vi "Tek_Read.vi"(8 "error in (no error)":errorcluster, 11 "VISA Refnum in":refnum<visa-resource-name>) -> (0 "error out":errorcluster, 1 "range":T1, 2 "Scope":cluster{dbl, dbl, dbl[]}(graph), 3 "VISA Refnum out":refnum<visa-resource-name>)   [LabVIEW 2022 SP3]
panel:
  out "data":dbl[](array[numeric])
  out "YOffset":dbl
  out "XZero":dbl
  out "YZero":dbl
  out "YMult":dbl
  out "XMult":dbl
  out "s/div":dbl
  out "V/div":dbl
  out "array":string[](array[string])
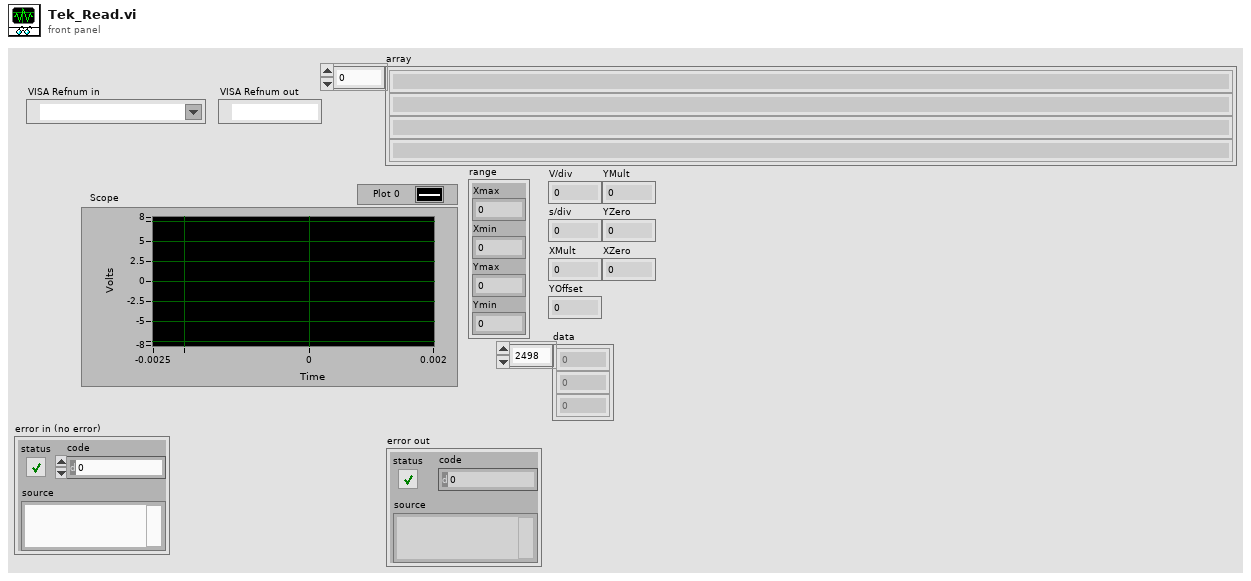
[diagram p1: front panel]
types:
  T1 = cluster{"Xmax":dbl, "Xmin":dbl, "Ymax":dbl, "Ymin":dbl}
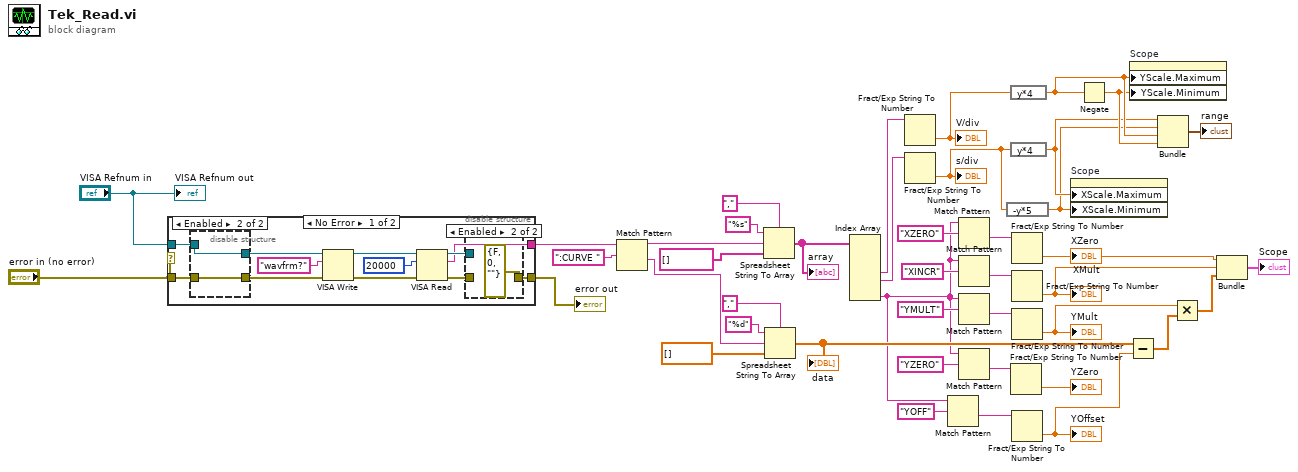
[diagram p0: block diagram]
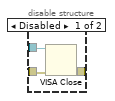
[diagram p2: hidden frame]
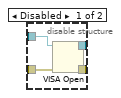
[diagram p3: hidden frame]
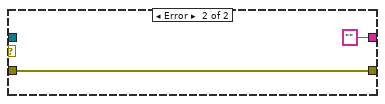
[diagram p4: hidden frame]
diagram:
  n1 = case shown="No Error" "error in (no error)" {
    tunnel: [w47 w67] -> w1
    tunnel: [w44 "" ("read buffer")] -> w41
    tunnel: "VISA Refnum in" -> [w50 _]
    tunnel: "error in (no error)" -> [w51 w67]
    frame No Error {
      n2 = disable-structure shown="Enabled" {
        disable-tunnel: w51 -> [w63 w64]
        disable-tunnel: w50 -> [w62 w65]
        disable-tunnel: [w61 w64] -> w49
        disable-tunnel: [w60 w65] -> w48
        frame Disabled {
          n3 = VISA Open(error in (no error)=w63, VISA resource name=w62) -> (VISA resource name=w60:refnum<visa-resource-name>, error out=w61:errorcluster)  [unwired: 3 in]
        }
        frame Enabled {
        }
      }
      n4 = VISA Write(VISA resource name=w48, write buffer="wavfrm?", error in (no error)=w49) -> (VISA resource name out=w54:refnum<visa-resource-name>, error out=w53:errorcluster)  [unwired: 1 out]
      n5 = VISA Read(VISA resource name=w54, byte count=u32 20000, error in (no error)=w53) -> (VISA resource name out=w45:refnum<visa-resource-name>, read buffer=w44:string, error out=w46:errorcluster)  [unwired: 1 out]
      n6 = disable-structure shown="Enabled" {
        disable-tunnel: [w58 errorcluster {"status"=FALSE, "code"=0, "source"=""} ("error out")] -> w47
        disable-tunnel: w46 -> [w57 _]
        disable-tunnel: w45 -> [w56 _]
        frame Disabled {
          n7 = VISA Close(VISA resource name=w56, error in (no error)=w57) -> (error out=w58:errorcluster)
        }
        frame Enabled {
        }
      }
    }
    frame Error {
    }
  }
  "error out" <- w1
  n8 = Match Pattern(string=w41, regular expression=":CURVE ") -> (before substring=w9:string, after substring=w8:string)  [unwired: 1 in, 2 out]
  n9 = Spreadsheet String To Array(delimiter (Tab)=",", format string="%s", spreadsheet string=w9, array type (2D Dbl)=string[] []) -> (array=w34:string[])
  "array" <- w34
  n10 = Spreadsheet String To Array(delimiter (Tab)=",", format string="%d", spreadsheet string=w8, array type (2D Dbl)=dbl[] []) -> (array=w23:dbl[])
  "data" <- w23
  n11 = Index Array(array=w34) -> (element #3=w33:string, element #4=w32:string, element #6=w14:string)  [unwired: 6 in, 3 out]
  n12 = Fract/Exp String To Number(string=w33) -> (number=w12:dbl)  [unwired: 3 in, 1 out]
  "V/div" <- w12
  n13 = Fract/Exp String To Number(string=w32) -> (number=w11:dbl)  [unwired: 3 in, 1 out]
  "s/div" <- w11
  n14 = Match Pattern(string=w14, regular expression="YOFF") -> (after substring=w16:string)  [unwired: 1 in, 3 out]
  n15 = Match Pattern(string=w14, regular expression="XZERO") -> (after substring=w25:string)  [unwired: 1 in, 3 out]
  n16 = Match Pattern(string=w14, regular expression="XINCR") -> (after substring=w30:string)  [unwired: 1 in, 3 out]
  n17 = Match Pattern(string=w14, regular expression="YMULT") -> (after substring=w29:string)  [unwired: 1 in, 3 out]
  n18 = Match Pattern(string=w14, regular expression="YZERO") -> (after substring=w26:string)  [unwired: 1 in, 3 out]
  n19 = expression code="-y*5"(w11) -> (w3:dbl)
  n20 = expression code="y*4"(w12) -> (w6:dbl)
  n21 = expression code="y*4"(w11) -> (w4:dbl)
  n22 = Fract/Exp String To Number(string=w26) -> (number=→"YZero":dbl)  [unwired: 3 in, 1 out]
  n23 = Fract/Exp String To Number(string=w25) -> (number=w19:dbl)  [unwired: 3 in, 1 out]
  "XZero" <- w19
  n24 = Fract/Exp String To Number(string=w30) -> (number=w18:dbl)  [unwired: 3 in, 1 out]
  "XMult" <- w18
  n25 = Fract/Exp String To Number(string=w29) -> (number=w20:dbl)  [unwired: 3 in, 1 out]
  "YMult" <- w20
  n26 = Fract/Exp String To Number(string=w16) -> (number=w13:dbl)  [unwired: 3 in, 1 out]
  "YOffset" <- w13
  n27 = property on="Scope" class="WFGraph (strict)"("XScale.Maximum"=w4, "XScale.Minimum"=w3) -> ()  [unwired: 2 in, 2 out]
  n28 = Negate(x=w6) -> (-x=w5:dbl)
  n29 = Subtract(x=w23, y=w13) -> (x-y=w21:dbl[])
  n30 = property on="Scope" class="WFGraph (strict)"("YScale.Maximum"=w6, "YScale.Minimum"=w5) -> ()  [unwired: 2 in, 2 out]
  n31 = Bundle(w4, w3, w6, w5) -> (→"range":cluster{dbl, dbl, dbl, dbl})  [unwired: 1 in]
  n32 = Multiply(x=w20, y=w21) -> (x*y=w17:dbl[])
  n33 = Bundle(w19, w18, w17) -> (→"Scope":cluster{dbl, dbl, dbl[]})  [unwired: 1 in]
  "VISA Refnum out" <- "VISA Refnum in"
